vi "Shell_Compare.vi"() -> ()   [LabVIEW 2019, in "lv-providershell-example1.lvlib"]
uses:
  lv-providershell-example1.lvlib
  LvProviderShellHelper/LvProviderShellHelper.lvclass
panel:
  out "Matched":bool
  out "error out":errorcluster
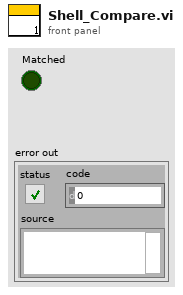
[diagram p1: front panel]
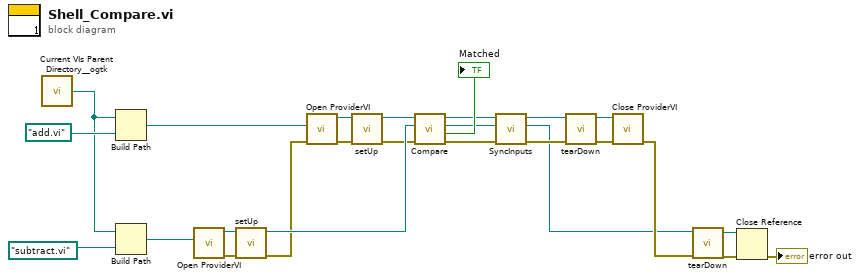
[diagram p0: block diagram]
diagram:
  n1 = call <userlib>:"Current VIs Parent Directory__ogtk.vi"() -> ("Parent Directory (+ Relative)"=w3:path)  [unwired: 5 in]
  n2 = Build Path(base path=w3, name or relative path=path "add.vi" ("vi path")) -> (appended path=w2:path)
  n3 = Build Path(base path=w3, name or relative path=path "subtract.vi" ("vi path")) -> (appended path=w1:path)
  n4 = call "Open ProviderVI.vi"("vi path"=w1) -> ("error out"=w23:errorcluster, "vi reference"=w24:refnum<vi>)  [unwired: 9 in]
  n5 = call "setUp.vi"("error in (no error)"=w23, "VI in"=w24) -> ("error out"=w20:errorcluster, "fpMgr out"=w21:refnum<class "LvProviderShellHelper.lvclass">)  [unwired: 8 in]
  n6 = call "Open ProviderVI.vi"("error in (no error)"=w20, "vi path"=w2) -> ("error out"=w25:errorcluster, "vi reference"=w26:refnum<vi>)  [unwired: 8 in]
  n7 = call "setUp.vi"("error in (no error)"=w25, "VI in"=w26) -> ("error out"=w19:errorcluster, "fpMgr out"=w22:refnum<class "LvProviderShellHelper.lvclass">)  [unwired: 8 in]
  n8 = call "Compare.vi"("error in (no error)"=w19, "fpMgr in"=w21, "Shell in"=w22) -> ("error out"=w10:errorcluster, "Matched"=→"Matched":bool, "fpMgr out"=w7:refnum<class "LvProviderShellHelper.lvclass">, "Shell out"=w11:refnum<class "LvProviderShellHelper.lvclass">)  [unwired: 5 in]
  n9 = call "SyncInputs.vi"("error in (no error)"=w10, "fpMgr in"=w7, "Shell in"=w11) -> ("error out"=w9:errorcluster, "fpMgr out"=w6:refnum<class "LvProviderShellHelper.lvclass">, "Shell out"=w8:refnum<class "LvProviderShellHelper.lvclass">)  [unwired: 6 in]
  n10 = call "tearDown.vi"("error in (no error)"=w9, "fpMgr in"=w8) -> ("error out"=w17:errorcluster, "VI"=w18:refnum<vi>)  [unwired: 8 in]
  n11 = call "Close ProviderVI.vi"("error in (no error)"=w17, "VI in"=w18) -> ("error out"=w16:errorcluster)  [unwired: 9 in]
  n12 = call "tearDown.vi"("error in (no error)"=w16, "fpMgr in"=w6) -> ("error out"=w14:errorcluster, "VI"=w15:refnum<vi>)  [unwired: 8 in]
  n13 = Close Reference(reference=w15, error in (no error)=w14) -> (error out=→"error out":errorcluster)
